vi "Pusher_Client_Utility_messageParser.vi"(8 "ErrIn":errorcluster, 11 "message":string="{\"event\":\"Mod1\",\"data\":\"{AI0:1.5,AI1:2.5,AI2:3.5,AI3:4.5}\",\"channel\":\"cRIO1\"}") -> (0 "ErrOut":errorcluster, 1 "data":cluster{"name":string, "value":string}[](array[cluster]), 2 "Channel":string, 3 "Event":string, 4 "RemainingData":string)   [LabVIEW 2009, in "Client.lvclass"]
uses:
  Client.lvclass
panel:
  # "Since there is no native JSON parser for LabVIEW, we have to\nstick to known format to pack our data while publishing it.\n\nFor this library,  data messages must be of the following format \n(key value json pairs) like\n\n{\"sampleRate\": \"1000\", \"message_count\": \"23\",\"message\":\"init\"}"
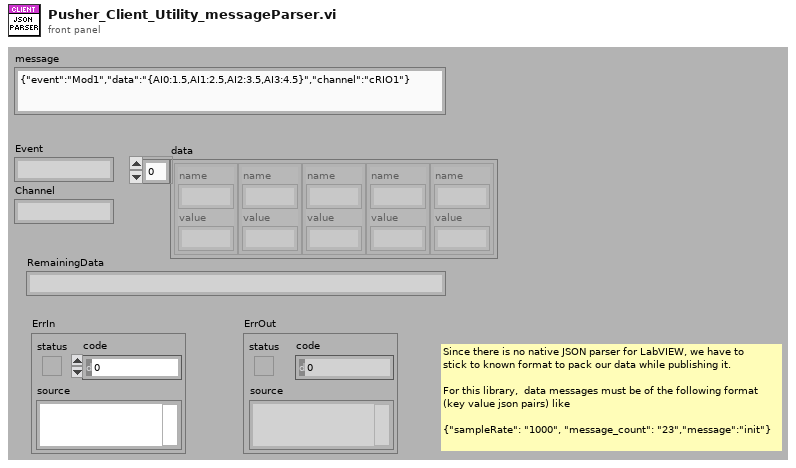
[diagram p1: front panel]
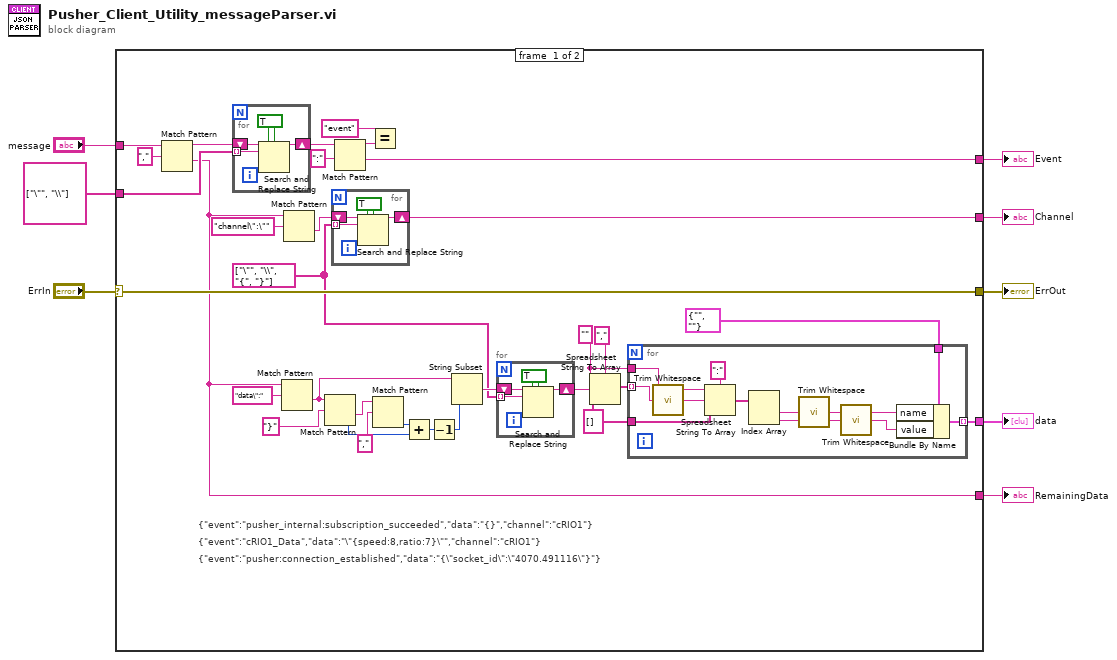
[diagram p0: block diagram]
diagram:
  n1 = case shown="No Error" "ErrIn" {
    selector: "ErrIn" -> [w40 w65]
    tunnel: [w40 w65] -> w7
    tunnel: "message" -> [w33 _]
    tunnel: [w34 _] -> w5
    tunnel: string[] ["\"", "\\"] -> [w27 _]
    tunnel: [w11 _] -> w3
    tunnel: [w10 _] -> w2
    tunnel: [w9 _] -> w1
    frame #0 {
      w16 = string[] ["\"", "\\", "{", "}"]
      w14 = string[] [] ("array type (2D Dbl)")
      w13 = "" ("format string")
      # "{\"event\":\"pusher:connection_established\",\"data\":\"{\\\"socket_id\\\":\\\"4070.491116\\\"}\"}"
      # "{\"event\":\"cRIO1_Data\",\"data\":\"\\\"{speed:8,ratio:7}\\\"\",\"channel\":\"cRIO1\"}"
      # "{\"event\":\"pusher_internal:subscription_succeeded\",\"data\":\"{}\",\"channel\":\"cRIO1\"}"
      n2 = Match Pattern(string=w33, regular expression=",") -> (before substring=w31:string, after substring=w9:string)  [unwired: 1 in, 2 out]
      n3 = for {
        shift-right: [w50] -> w30
        shift-left: w31 -> [w52]
        tunnel: w27 -> [w49] mode=indexing
        w51 = TRUE ("replace all? (F)")
        n4 = Search and Replace String(replace all?=w51, case sensitive?=w51, input string=w52, search string=w49) -> (result string=w50:string)  [unwired: 4 in, 3 out]
      }
      n5 = Match Pattern(string=w9, regular expression="data\":") -> (after substring=w20:string)  [unwired: 1 in, 3 out]
      n6 = Match Pattern(string=w9, regular expression="channel\":\"") -> (after substring=w28:string)  [unwired: 1 in, 3 out]
      n7 = Match Pattern(string=w20, regular expression="}") -> (after substring=w23:string, offset past match=w21:i32)  [unwired: 1 in, 2 out]
      n8 = for {
        shift-right: [w46] -> w10
        shift-left: w28 -> [w48]
        tunnel: w16 -> [w45] mode=indexing
        w47 = TRUE ("replace all? (F)")
        n9 = Search and Replace String(replace all?=w47, case sensitive?=w47, input string=w48, search string=w45) -> (result string=w46:string)  [unwired: 4 in, 3 out]
      }
      n10 = Match Pattern(string=w30, regular expression=":") -> (before substring=w36:string, after substring=w34:string)  [unwired: 1 in, 2 out]
      n11 = Equal?(x="event", y=w36) -> ()  [unwired: 1 out]
      n12 = Match Pattern(string=w23, regular expression=",") -> (offset past match=w22:i32)  [unwired: 1 in, 3 out]
      n13 = Add(x=w22, y=w21) -> (x+y=w19:i32)
      n14 = Decrement(x=w19) -> (x-1=w18:i32)
      n15 = String Subset(string=w20, length (rest)=w18) -> (substring=w17:string)  [unwired: 1 in]
      n16 = for {
        shift-right: [w42] -> w15
        shift-left: w17 -> [w44]
        tunnel: w16 -> [w41] mode=indexing
        w43 = TRUE ("replace all? (F)")
        n17 = Search and Replace String(replace all?=w43, case sensitive?=w43, input string=w44, search string=w41) -> (result string=w42:string)  [unwired: 4 in, 3 out]
      }
      n18 = Spreadsheet String To Array(delimiter (Tab)=",", format string=w13, spreadsheet string=w15, array type (2D Dbl)=w14) -> (array=w38:string[])
      n19 = for {
        tunnel: w38 -> [w64] mode=indexing
        tunnel: w14 -> [w63]
        tunnel: w13 -> [w62]
        tunnel: cluster{"name":string, "value":string} {"name"="", "value"=""} -> [w59]
        tunnel: [w56] -> w11 mode=indexing
        n20 = call <vilib>:"Trim Whitespace.vi"("string"=w64) -> ("trimmed string"=w53:string)  [unwired: 1 in]
        n21 = Spreadsheet String To Array(delimiter (Tab)=":", format string=w62, spreadsheet string=w53, array type (2D Dbl)=w63) -> (array=w60:string[])
        n22 = Index Array(array=w60) -> (element #1=w58:string, element #2=w57:string)  [unwired: 2 in]
        n23 = call <vilib>:"Trim Whitespace.vi"("string"=w58) -> ("trimmed string"=w55:string)  [unwired: 1 in]
        n24 = call <vilib>:"Trim Whitespace.vi"("string"=w57) -> ("trimmed string"=w54:string)  [unwired: 1 in]
        n25 = Bundle By Name(cluster=w59, "name"=w55, "value"=w54) -> (w56:cluster{"name":string, "value":string})
      }
    }
    frame #1 {
    }
  }
  "ErrOut" <- w7
  "Event" <- w5
  "data" <- w3
  "Channel" <- w2
  "RemainingData" <- w1
